vi "Angle_M_v2.vi"() -> ()   [LabVIEW 2024]
panel:
  out "Array":string[](array[string])
  in  "Select File":bool
  in  "Plot":bool
  out "new picture":picture
  out "before substring":string
  in  "stop":bool
  out "error out":errorcluster
  out "standard output":string
  out "standard error":string
  in  "Path":path
  out "Count":i32
  out "current time":timestamp
  in  "milliseconds to wait":u32
  out "Ping":errorcluster
  out "Ping Error":string
  out "Ping Output":string
  out "error out 3":errorcluster
  out "Server Error":string
  out "Server Output":string
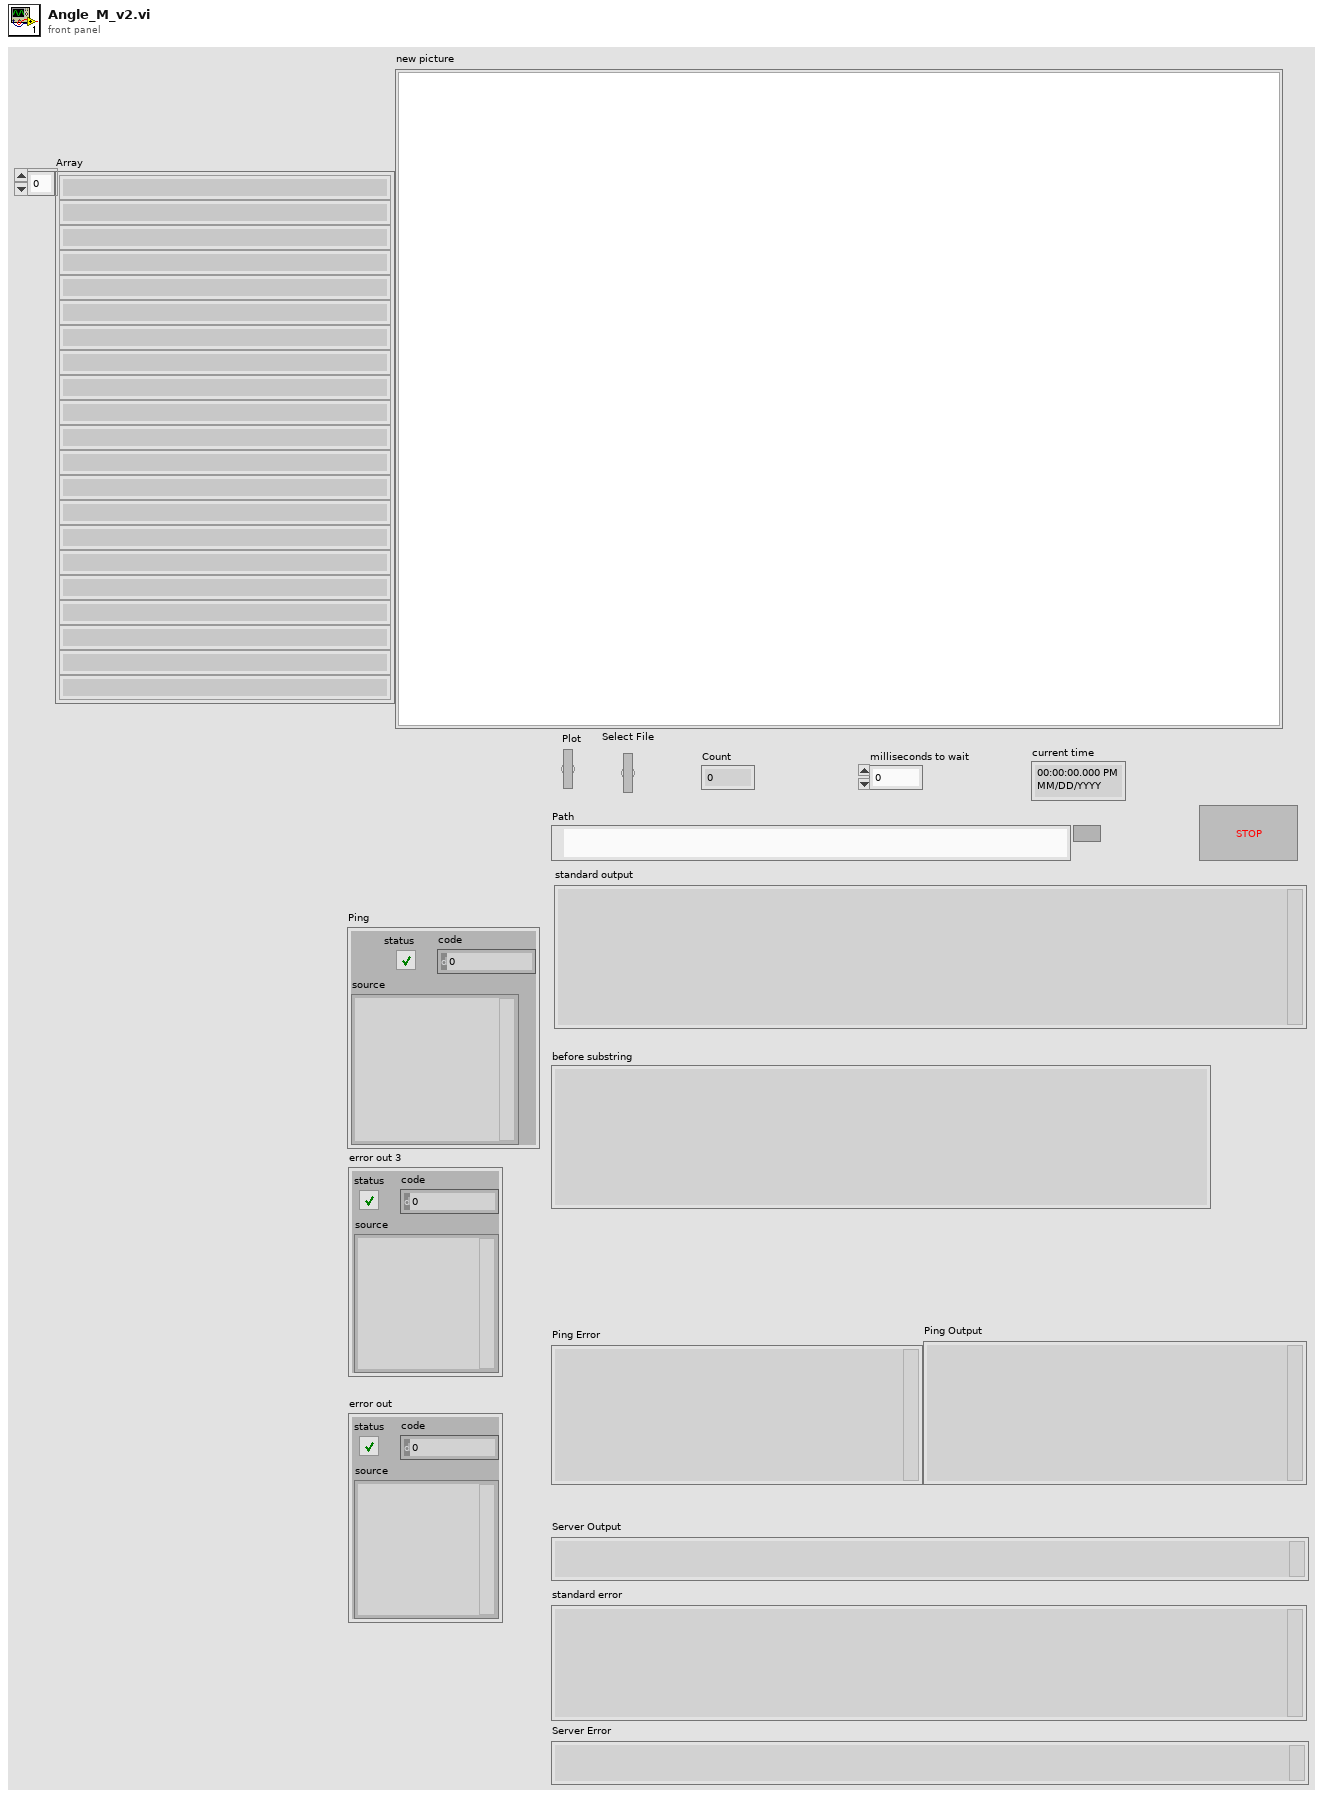
[diagram p1: front panel]
types:
  T1 = typedef "imagedata.ctl" = cluster{"image type":i32, "image depth":i32, "image":u8[], "mask":u8[], "colors":u32[], "Rectangle":cluster{"left":i16, "top":i16, "right":i16, "bottom":i16}}
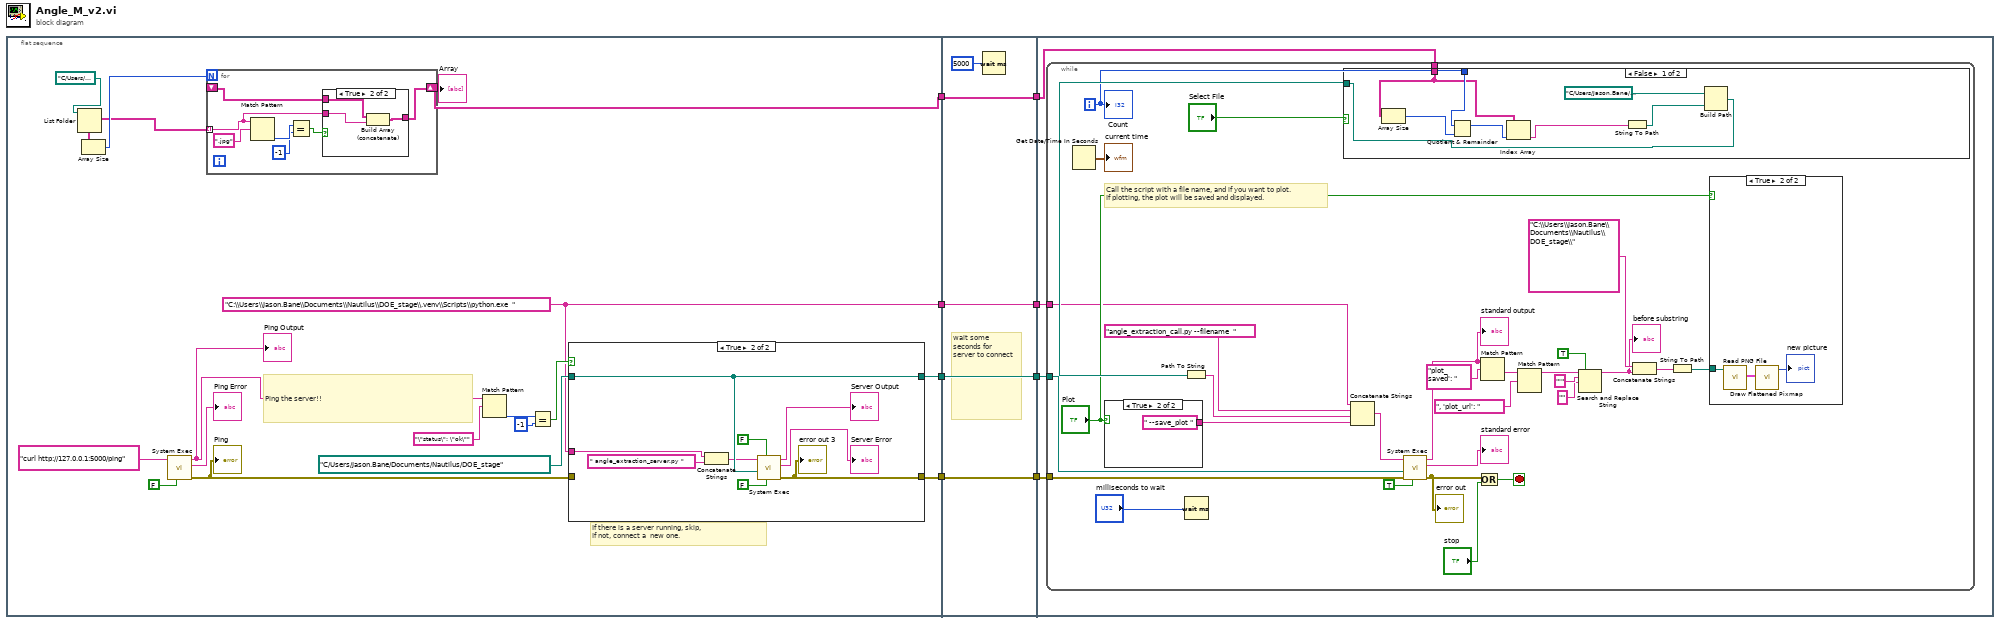
[diagram p0: block diagram]
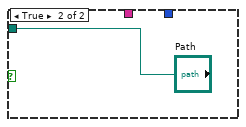
[diagram p4: hidden frame]
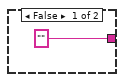
[diagram p6: hidden frame]
diagram:
  n1 = flat-sequence {
    tunnel: [w22] -> w8
    tunnel: [w21] -> w6
    tunnel: [w13] -> w3
    tunnel: [w10] -> w1
    tunnel: w8 -> [w52]
    tunnel: [w52] -> w7
    tunnel: w6 -> [w51]
    tunnel: [w51] -> w5
    tunnel: [w49] -> w4
    tunnel: w3 -> [w49]
    tunnel: [w48] -> w2
    tunnel: w1 -> [w48]
    tunnel: w7 -> [w56]
    tunnel: w5 -> [w55]
    tunnel: w4 -> [w54]
    tunnel: w2 -> [w53]
    frame #0 {
      w13 = "C:\\Users\\Jason.Bane\\Documents\\Nautilus\\DOE_stage\\.venv\\Scripts\\python.exe  "
      # "If there is a server running, skip,\nIf not, connect a  new one."
      # "Ping the server!!"
      n2 = List Folder(path=path "C:/Users/Jason.Bane/Documents/Nautilus/DOE_stage/code_trials/images") -> (filenames=w9:string[])  [unwired: 3 in, 3 out]
      n3 = Array Size(array=w9) -> (size(s)=w11:i32)
      n4 = call <vilib>:"System Exec.vi"("run minimized? (F)"=FALSE, "command line"="curl http://127.0.0.1:5000/ping") -> ("error out"=w14:errorcluster, "standard error"=→"Ping Error":string, "standard output"=w19:string)  [unwired: 6 in, 1 out]
      "Ping Output" <- w19
      "Ping" <- w14
      n5 = for {
        N: w11 -> [_]
        tunnel: w9 -> [w28] mode=indexing
        shift-right: [w27] -> w10
        shift-left: _ -> [w26]
        n6 = Match Pattern(string=w28, regular expression=".jpg") -> (offset past match=w31:i32)  [unwired: 1 in, 3 out]
        n7 = Equal?(x=w31, y=-1) -> (x = y?=w29:bool)
        n8 = case shown="True" w29 {
          tunnel: w28 -> [_ w36]
          tunnel: [w33 w35] -> w27
          tunnel: w26 -> [w33 w34]
          frame False {
          }
          frame True {
            n9 = Build Array (concatenate)(w34, w36) -> (w35:string[])
          }
        }
      }
      "Array" <- w10
      n10 = Match Pattern(string=w19, regular expression="\"status\": \"ok\"") -> (offset past match=w17:i32)  [unwired: 1 in, 3 out]
      n11 = Equal?(x=w17, y=-1) -> (x = y?=w15:bool)
      n12 = case shown="True" w15 {
        tunnel: [w38 w43] -> w21
        tunnel: [w37 w44] -> w22
        tunnel: path "C:/Users/Jason.Bane/Documents/Nautilus/DOE_stage" ("working directory") -> [w38 w43]
        tunnel: w14 -> [w37 _]
        tunnel: w13 -> [_ w41]
        frame False {
        }
        frame True {
          n13 = Concatenate Strings(w41, " angle_extraction_server.py " ("command line")) -> (w39:string)
          n14 = call <vilib>:"System Exec.vi"("run minimized? (F)"=FALSE, "wait until completion? (T)"=FALSE, "working directory"=w43, "command line"=w39) -> ("error out"=w44:errorcluster, "standard error"=→"Server Error":string, "standard output"=→"Server Output":string)  [unwired: 4 in, 1 out]
          "error out 3" <- w44
        }
      }
    }
    frame #1 {
      # "wait some  seconds for \nserver to connect"
      n15 = Wait (ms)(milliseconds to wait=u32 5000) -> ()  [unwired: 1 out]
    }
    frame #2 {
      n16 = while {
        tunnel: w55 -> [w79]
        tunnel: w56 -> [w78]
        tunnel: w54 -> [w60]
        tunnel: w53 -> [w57]
        i -> [w58]
        stop <- w87 stop-if-true
        # "Call the script with a file name, and if you want to plot. \nIf plotting, the plot will be saved and displayed."
        n17 = Get Date/Time In Seconds() -> (seconds since 1Jan1904=→"current time":timestamp)
        n18 = case shown="True" "Plot" {
          tunnel: ["" " --save_plot "] -> w63
          frame False {
          }
          frame True {
          }
        }
        n19 = Wait (ms)(milliseconds to wait="milliseconds to wait") -> ()  [unwired: 1 out]
        n20 = case shown="False" "Select File" {
          tunnel: [w88 "Path"] -> w82
          tunnel: w58 -> [w95 _]
          tunnel: w57 -> [w93 _]
          frame False {
            n21 = Array Size(array=w93) -> (size(s)=w94:i32)
            n22 = Quotient & Remainder(x=w95, y=w94) -> (x-y*floor(x/y)=w92:i32)  [unwired: 1 out]
            n23 = Index Array(array=w93, index=w92) -> (element=w91:string)
            n24 = String To Path(string=w91) -> (path=w89:path)
            n25 = Build Path(base path=path "C:/Users/Jason.Bane/Documents/Nautilus/DOE_stage/code_trials/images", name or relative path=w89) -> (appended path=w88:path)
          }
          frame True {
          }
        }
        n26 = Path To String(path=w82) -> (string=w81:string)
        n27 = Concatenate Strings(w60, "angle_extraction_call.py --filename  ", w81, w63) -> (w80:string)
        n28 = call <vilib>:"System Exec.vi"("run minimized? (F)"=TRUE, "error in (no error)"=w78, "working directory"=w79, "command line"=w80) -> ("error out"=w85:errorcluster, "standard error"=→"standard error":string, "standard output"=w75:string)  [unwired: 4 in, 1 out]
        "error out" <- w85
        "standard output" <- w75
        n29 = Or(x=w85, y="stop") -> (x .or. y?=w87:bool)
        n30 = Match Pattern(string=w75, regular expression="plot_saved': ") -> (after substring=w71:string)  [unwired: 1 in, 3 out]
        n31 = Match Pattern(string=w71, regular expression=", 'plot_url': ") -> (before substring=w69:string)  [unwired: 1 in, 3 out]
        n32 = Search and Replace String(replace all?=TRUE ("replace all? (F)"), input string=w69, search string="'", replace string="" ("replace string (\"\")")) -> (result string=w66:string)  [unwired: 4 in, 3 out]
        "before substring" <- w66
        n33 = Concatenate Strings("C:\\Users\\Jason.Bane\\Documents\\Nautilus\\DOE_stage\\" ("string"), w66) -> (w64:string)
        n34 = String To Path(string=w64) -> (path=w72:path)
        n35 = case shown="True" "Plot" {
          tunnel: w72 -> [_ w99]
          frame False {
          }
          frame True {
            n36 = call <vilib>:"Read PNG File.vi"("path to PNG file"=w99) -> ("image data"=w98:T1)  [unwired: 8 in, 2 out]
            n37 = call <vilib>:"Draw Flattened Pixmap.vi"("image data"=w98) -> ("new picture"=→"new picture":picture)  [unwired: 8 in]
          }
        }
        "Count" <- w58
      }
    }
  }
